vi "To XML.vi"(8 "error in (no error)":errorcluster, 9 "Parent":refnum<k20>, 10 "Document":refnum<k20>, 11 "Line in":refnum<class "Line.lvclass">) -> (0 "error out":errorcluster)   [LabVIEW 2017, in "Cobertura.lvlib" / "Line.lvclass"]
uses:
  Line.lvclass
  Line.lvclass/Line.ctl
  <vilib>/xml/Close Reference(Node).vi
  <resource>/objmgr/DOMUserDefRef.rc
  <vilib>/xml/NI_XML.lvlib
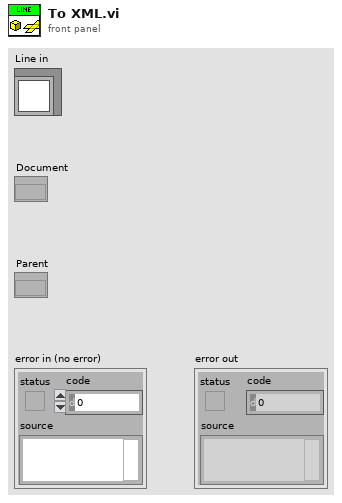
[diagram p1: front panel]
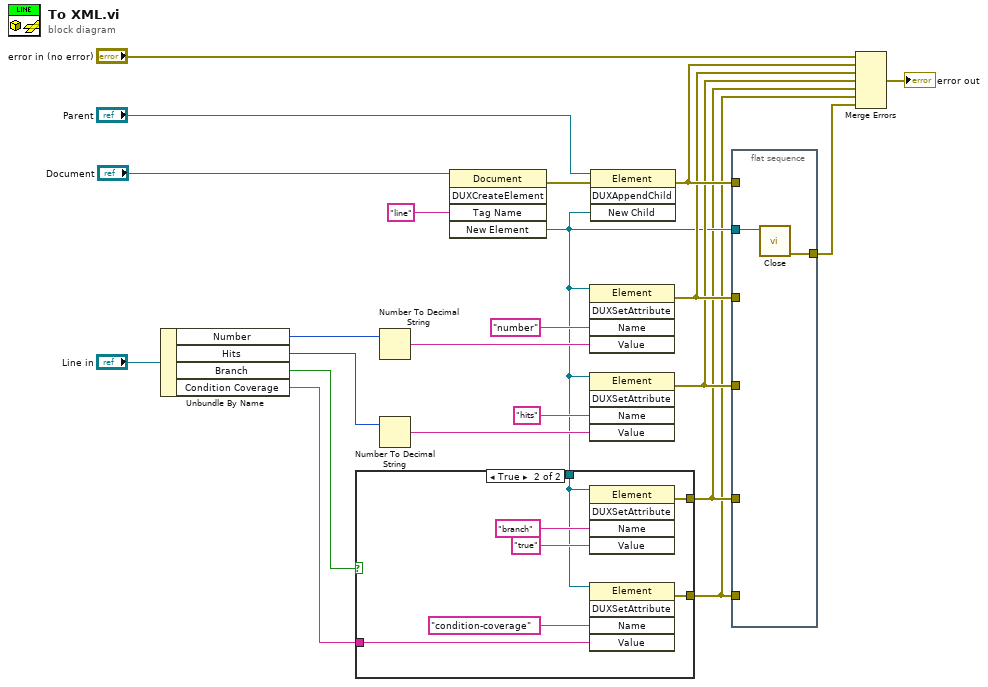
[diagram p0: block diagram]
diagram:
  n1 = Unbundle By Name("Line in") -> ("Number"=w15:u32, "Hits"=w18:u32, "Branch"=w1:bool, "Condition Coverage"=w4:string)
  n2 = Number To Decimal String(number=w15) -> (decimal integer string=w14:string)  [unwired: 1 in]
  n3 = Number To Decimal String(number=w18) -> (decimal integer string=w20:string)  [unwired: 1 in]
  n4 = invoke class="Document" method="DUXCreateElement"(reference="Document", "Tag Name"="line") -> (error out=w12:errorcluster, "New Element"=w5:refnum<k20>)  [unwired: 3 in, 3 out]
  n5 = case shown="True" w1 {
    tunnel: w5 -> [_ w26]
    tunnel: w4 -> [_ w25]
    tunnel: [_ w24] -> w3
    tunnel: [_ w23] -> w2
    frame False {
    }
    frame True {
      n6 = invoke class="Element" method="DUXSetAttribute"(reference=w26, "Name"="branch", "Value"="true" ("Name")) -> (error out=w24:errorcluster)  [unwired: 2 in, 4 out]
      n7 = invoke class="Element" method="DUXSetAttribute"(reference=w26, "Name"="condition-coverage", "Value"=w25) -> (error out=w23:errorcluster)  [unwired: 2 in, 4 out]
    }
  }
  n8 = invoke class="Element" method="DUXSetAttribute"(reference=w5, "Name"="number", "Value"=w14) -> (error out=w7:errorcluster)  [unwired: 2 in, 4 out]
  n9 = invoke class="Element" method="DUXSetAttribute"(reference=w5, "Name"="hits", "Value"=w20) -> (error out=w6:errorcluster)  [unwired: 2 in, 4 out]
  n10 = invoke class="Element" method="DUXAppendChild"(reference="Parent", error in=w12, "New Child"=w5) -> (error out=w8:errorcluster)  [unwired: 1 in, 3 out]
  n11 = flat-sequence {
    tunnel: w5 -> [w31]
    tunnel: [w30] -> w9
    tunnel: w8 -> [_]
    tunnel: w7 -> [_]
    tunnel: w6 -> [_]
    tunnel: w3 -> [_]
    tunnel: w2 -> [_]
    frame #0 {
      n12 = call-poly <vilib>:"Close.vi"("node"=w31) -> ("error out"=w30:errorcluster)  [unwired: 8 in]
    }
  }
  n13 = Merge Errors("error in (no error)", w8, w7, w6, w3, w2, w9) -> (→"error out":errorcluster)
